vi "Comments.Add Lockin Description.vi"(7 "error in (no error)":errorcluster, 10 "Control Experiment":refnum<class "Control Experiment.lvclass">) -> (0 "error out":errorcluster, 3 "Control Experiment out":refnum<class "Control Experiment.lvclass">)   [LabVIEW 2019, in "Control Experiment.lvclass"]
uses:
  Control Experiment.lvclass
  Control Experiment.lvclass/Control Experiment.ctl
  <userlib>/LevyLab/Lockin-Multichannel/Instrument.Lockin/Instrument.Lockin.lvclass
  <userlib>/LevyLab/PLYM/YAML.lvclass
panel:
  out "Lockin Comments":string
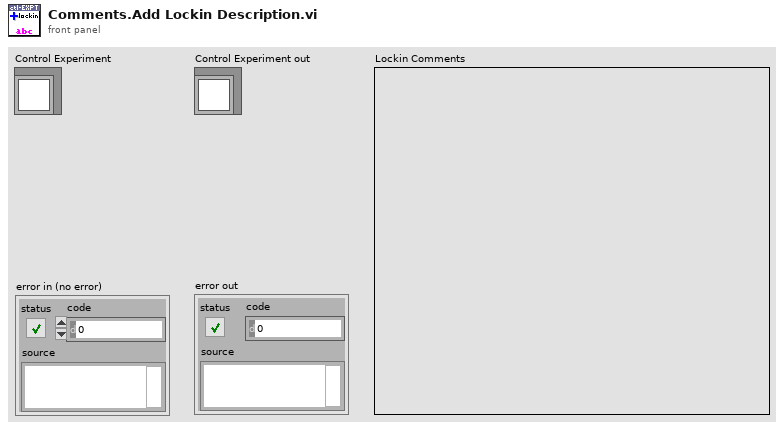
[diagram p1: front panel]
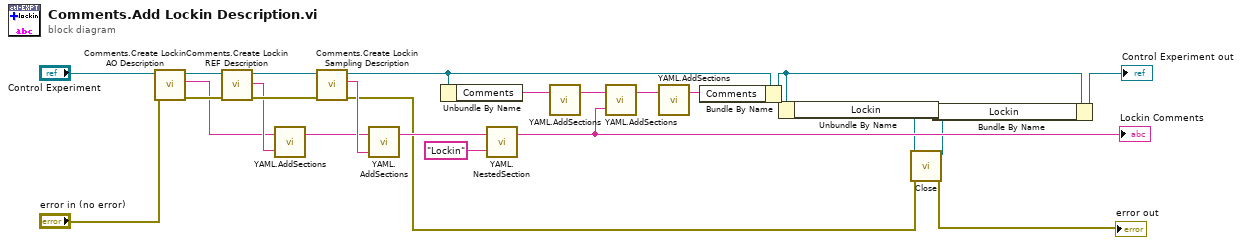
[diagram p0: block diagram]
diagram:
  n1 = call "Comments.Create Lockin AO Description.vi"("error in (no error)"="error in (no error)", "Control Experiment"="Control Experiment") -> ("error out"=w19:errorcluster, "AO Section"=w11:string, "Control Experiment out"=w20:refnum<class "Control Experiment.lvclass">)  [unwired: 6 in]
  n2 = call "Comments.Create Lockin REF Description.vi"("error in (no error)"=w19, "Control Experiment"=w20) -> ("error out"=w17:errorcluster, "REF Section"=w13:string, "Control Experiment out"=w18:refnum<class "Control Experiment.lvclass">)  [unwired: 6 in]
  n3 = call <userlib>:"YAML.AddSections.vi"("Section 2"=w13, "Section 1"=w11) -> ("Output"=w12:string)  [unwired: 1 in]
  n4 = call "Comments.Create Lockin Sampling Description.vi"("error in (no error)"=w17, "Control Experiment"=w18) -> ("error out"=w2:errorcluster, "Sampling Section"=w14:string, "Control Experiment out"=w21:refnum<class "Control Experiment.lvclass">)  [unwired: 6 in]
  n5 = call <userlib>:"YAML.AddSections.vi"("Section 2"=w14, "Section 1"=w12) -> ("Output"=w10:string)  [unwired: 1 in]
  n6 = Unbundle By Name(w21) -> ("Comments"=w24:string)
  n7 = call <userlib>:"YAML.NestedSection.vi"("Section Key"="Lockin" ("string"), "Nested Section"=w10) -> ("String"=w15:string)  [unwired: 1 in]
  "Lockin Comments" <- w15
  n8 = call <userlib>:"YAML.AddSections.vi"("Section 1"=w24) -> ("Output"=w23:string)  [unwired: 2 in]
  n9 = call <userlib>:"YAML.AddSections.vi"("Section 2"=w15, "Section 1"=w23) -> ("Output"=w8:string)  [unwired: 1 in]
  n10 = call <userlib>:"YAML.AddSections.vi"("Section 1"=w8) -> ("Output"=w7:string)  [unwired: 2 in]
  n11 = Bundle By Name(cluster=w21, "Comments"=w7) -> (w6:refnum<class "Control Experiment.lvclass">)
  n12 = Unbundle By Name(w6) -> ("Lockin"=w4:refnum<class "Instrument.Lockin.lvclass">)
  n13 = call-dynamic "Close.vi"("error in (no error)"=w2, "Instrument.Lockin in"=w4) -> ("error out"=→"error out":errorcluster, "Instrument.Lockin out"=w3:refnum<class "Instrument.Lockin.lvclass">)  [unwired: 8 in]
  n14 = Bundle By Name(cluster=w6, "Lockin"=w3) -> (→"Control Experiment out":refnum<class "Control Experiment.lvclass">)
